vi "file_checkName.vi"(0 "path":path, 2 "filename extension":string, 5 "error in (no error)":errorcluster) -> (14 "path string out":string, 16 "actual path":path, 18 "exist":bool, 19 "error out":errorcluster)   [LabVIEW 2010, in "OSA.lvclass"]
doc: "SubVI to a <B>Thorlabs_OSA_64</B> object.\n\n[GOOP 1.0]"
uses:
  OSA.lvclass
  OSA20X_misc.lvlib
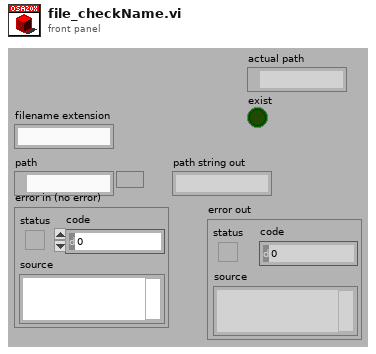
[diagram p1: front panel]
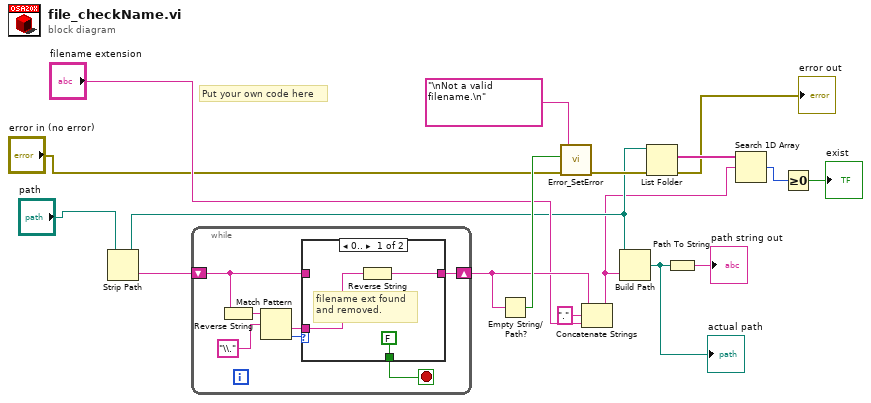
[diagram p0: block diagram]
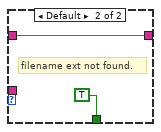
[diagram p2: hidden frame]
diagram:
  # "Put your own code here"
  n1 = Strip Path(path="path") -> (stripped path=w6:path, name=w13:string)
  n2 = while {
    shift-right: [w19] -> w12
    shift-left: w13 -> [w20]
    stop <- w18 stop-if-true
    n3 = Reverse String(1:w20) -> (0:w23:string)
    n4 = Match Pattern(string=w23, regular expression="\\.") -> (after substring=w21:string, offset past match=w22:i32)  [unwired: 1 in, 2 out]
    n5 = case shown="0.." w22 {
      tunnel: w20 -> [_ w29]
      tunnel: [w26 w29] -> w19
      tunnel: w21 -> [w27 _]
      tunnel: [FALSE TRUE] -> w18
      frame 0.. {
        # "filename ext found\nand removed."
        n6 = Reverse String(1:w27) -> (0:w26:string)
      }
      frame Default {
        # "filename ext not found."
      }
    }
  }
  n7 = Empty String/Path?(string/path=w12) -> (empty?=w15:bool)
  n8 = call "Error_SetError.vi"("error in"="error in (no error)", "status (true)"=w15, "source(\"\")"="\nNot a valid filename.\n" ("source(\"\")")) -> ("error out"=w7:errorcluster)  [unwired: 4 in]
  n9 = Concatenate Strings(w12, "." ("string"), "filename extension") -> (w4:string)
  n10 = Build Path(base path=w6, name or relative path=w4) -> (appended path=w17:path)
  "actual path" <- w17
  n11 = List Folder(path=w6, error in=w7) -> (filenames=w5:string[], error out=→"error out":errorcluster)  [unwired: 2 in, 2 out]
  n12 = Path To String(path=w17) -> (string=→"path string out":string)
  n13 = Search 1D Array(1D array=w5, element=w4) -> (index of element=w2:i32)  [unwired: 1 in]
  n14 = Greater Or Equal To 0?(x=w2) -> (x >= 0?=→"exist":bool)
